vi "SV Multitone SINAD and THD+N (Frequency) (1 Ch).vi"(0 "complex spectrum response":T9={"complex spectrum response"={"f0"=0.0, "df"=1.0, "complex spectrum"=[]}, "spectrum info"={"channel name"="", "description"="", "x-axis units"=0, "spectral info"={"spectrum type"=enum."Power [Magnitude^2]", "linear/dB"=enum."linear", "window"=0, "window size"=0, "FFT size"=0}, "engineering units"=0, "custom label"="", "dB reference [EU]"=0.0, "peak units"=enum."rms", "weighting filter"=0, "spectral density?"=FALSE, "unit label"="", "spectrum skewed?"=FALSE, "complimentary spectrum units"=enum."none"}} {"spectrum info"."x-axis units" items=["Time (s)"=0, "Frequency-CB (Hz)"=1, "Frequency-CPB (Hz)"=1248, "Frequency-Arbitrary (Hz)"=2357, "Quefrency (s)"=2, "Revolutions (rev)"=3, "Order"=4, "Speed (RPM)"=11, "Speed (rad/s)"=21, "Index"=65535]; "spectrum info"."weighting filter" items=["Linear", "A-weighting", "B-weighting", "C-weighting", "ITU-R 468-4", "Dolby", "CCITT", "C-message", "Wb", "Wc", "Wd", "We", "Wf", "Wh", "Wj", "Wk", "Wm", "AES17 20 kHz lowpass", "AES17 40 kHz lowpass", "AES17 20 kHz highpass", "AES17 40 kHz highpass"]; "spectrum info"."dB reference [EU]" format="%.2f"; "spectrum info"."engineering units" items=["custom..."=0, "V"=1, "A"=21, "C"=30, "pC"=31, "s"=32, "-"=29, "Pa"=2, "N"=20, "g"=3, "m/s^2"=4, "m/s"=5, "m"=6, "mm/s"=12, "mm"=13, "micron/s"=14, "micron"=15, "in/s^2"=7, "in/s"=8, "in"=9, "mil/s"=10, "mil"=11, "rad/s^2"=16, "rad/s"=17, "rad"=18, "deg/s^2"=26, "deg/s"=27, "deg"=28, "RPM"=22, "cycle/s^2"=23, "Hz"=24, "cycle"=25, "strain"=19]; "spectrum info"."spectral info"."window" items=["None "=0, "Hanning"=1, "Hamming"=2, "Blackman-Harris"=3, "Exact Blackman"=4, "Blackman"=5, "Flat Top"=6, "4 Term B-Harris "=7, "7 Term B-Harris"=8, "Low Sidelobe"=9, "Force - Exponential"=10, "Gaussian"=62]; "complex spectrum response"."complex spectrum" format="%.2f"; "complex spectrum response"."df" format="%.2f"; "complex spectrum response"."f0" format="%.2f"}, 1 "reference tones":T2(array[cluster]) {"phase (deg)" format="%0.3p"; "amplitude [EU pk]" format="%0.3p"; "frequency [Hz]" format="%0.3p"}, 2 "frequency range":T11={"start frequency"=-1.0, "stop frequency"=-1.0} {"stop frequency" format="%.2f"; "start frequency" format="%.2f"}, 3 "advanced span [Hz]":dbl=-1.0 format="%.2f", 5 "error in (no error)":errorcluster, 6 "desired units":T12={"SINAD"=enum."dB", "THD+N"=enum."dB", "response level"=enum."EU rms", "noise and distortion level"=enum."EU rms"}) -> (12 "unit labels":T10, 14 "complex spectrum response":T9={"complex spectrum response"={"f0"=0.0, "df"=1.0, "complex spectrum"=[]}, "spectrum info"={"channel name"="", "description"="", "x-axis units"=0, "spectral info"={"spectrum type"=enum."Power [Magnitude^2]", "linear/dB"=enum."linear", "window"=0, "window size"=0, "FFT size"=0}, "engineering units"=0, "custom label"="", "dB reference [EU]"=0.0, "peak units"=enum."rms", "weighting filter"=0, "spectral density?"=FALSE, "unit label"="", "spectrum skewed?"=FALSE, "complimentary spectrum units"=enum."none"}} {"spectrum info"."x-axis units" items=["Time (s)"=0, "Frequency-CB (Hz)"=1, "Frequency-CPB (Hz)"=1248, "Frequency-Arbitrary (Hz)"=2357, "Quefrency (s)"=2, "Revolutions (rev)"=3, "Order"=4, "Speed (RPM)"=11, "Speed (rad/s)"=21, "Index"=65535]; "spectrum info"."weighting filter" items=["Linear", "A-weighting", "B-weighting", "C-weighting", "ITU-R 468-4", "Dolby", "CCITT", "C-message", "Wb", "Wc", "Wd", "We", "Wf", "Wh", "Wj", "Wk", "Wm", "AES17 20 kHz lowpass", "AES17 40 kHz lowpass", "AES17 20 kHz highpass", "AES17 40 kHz highpass"]; "spectrum info"."dB reference [EU]" format="%.2f"; "spectrum info"."engineering units" items=["custom..."=0, "V"=1, "A"=21, "C"=30, "pC"=31, "s"=32, "-"=29, "Pa"=2, "N"=20, "g"=3, "m/s^2"=4, "m/s"=5, "m"=6, "mm/s"=12, "mm"=13, "micron/s"=14, "micron"=15, "in/s^2"=7, "in/s"=8, "in"=9, "mil/s"=10, "mil"=11, "rad/s^2"=16, "rad/s"=17, "rad"=18, "deg/s^2"=26, "deg/s"=27, "deg"=28, "RPM"=22, "cycle/s^2"=23, "Hz"=24, "cycle"=25, "strain"=19]; "spectrum info"."spectral info"."window" items=["None "=0, "Hanning"=1, "Hamming"=2, "Blackman-Harris"=3, "Exact Blackman"=4, "Blackman"=5, "Flat Top"=6, "4 Term B-Harris "=7, "7 Term B-Harris"=8, "Low Sidelobe"=9, "Force - Exponential"=10, "Gaussian"=62]; "complex spectrum response"."complex spectrum" format="%.2f"; "complex spectrum response"."df" format="%.2f"; "complex spectrum response"."f0" format="%.2f"}, 15 "SINAD":dbl format="%.2f", 16 "THD+N":dbl format="%.2f", 18 "levels":T1 {"noise and distortion" format="%.2f"; "response" format="%.2f"}, 19 "error out":errorcluster)   [LabVIEW 2017, in "SoundVib_Multitone.lvlib"]
doc: "Performs a total harmonic distortion plus noise (THD+N) analysis, including measuring the fundamental tone, and returns the detected fundamental frequency, detected fundamental amplitude, and THD+N. Signal in noise and distortion (SINAD) is the negative of THD+N in dB. Wire data to the<B> scaled signal [EU]</B> input to determine the polymorphic instance to use or manually select the instance.\n\nThe following formula calculates THD+N:\n\nTHD+N = sqrt(H^2 + N^2) / sqrt(F^2 + N^2 + H^2)\n\nwhere H is the harmonic RMS level, N is the noise RMS level, and F is the fundamental tone RMS level."
uses:
  <vilib>/addons/Sound and Vibration/svt_Multitone Distortion/SoundVib_Multitone.lvlib
  <vilib>/addons/_NISVFA/_Shared subVIs/Controls/svc_Spectrum Info.ctl
  <vilib>/addons/_NISVFA/_Shared subVIs/Controls/svc_X-Axis Units.ctl
  <vilib>/addons/_NISVFA/_Shared subVIs/Controls/svc_Spectrum Type.ctl
  <vilib>/addons/_NISVFA/_Shared subVIs/Controls/svc_Engineering Units Text Ring.ctl
  <vilib>/addons/_NISVFA/_Shared subVIs/Controls/svc_Weighting Filter Text Ring.ctl
  <vilib>/addons/_NISVFA/_Shared subVIs/Controls/svc_Complimentary Spectrum Units.ctl
  <vilib>/addons/_NISVFA/_Spectrum Processing/SVPO Power in Band (Complex) (1 Ch).vi
  <vilib>/Analysis/BLAS.llb/nrm2 - Vector 2-Norm.vi
  <vilib>/Analysis/BLAS.llb/dznrm2 - Vector 2-Norm (CDB).vi
  <vilib>/addons/_NISVFA/_Shared subVIs/Common/svc_Convert Start and Stop to Start Index and Length.vi
  <vilib>/addons/_NISVFA/_Shared subVIs/Common/svc_Window Parameters.vi
  <vilib>/addons/_NISVFA/_Spectrum Processing/subVIs/svfa_Spectrum Info Window to windowTd Type Def.vi
  <vilib>/addons/_NISVFA/_Spectrum Processing/SVFA Get Spectrum Subset (Complex) (1 Ch).vi
  <vilib>/addons/Sound and Vibration/svt_Distortion/SoundVib_Distortion.lvlib
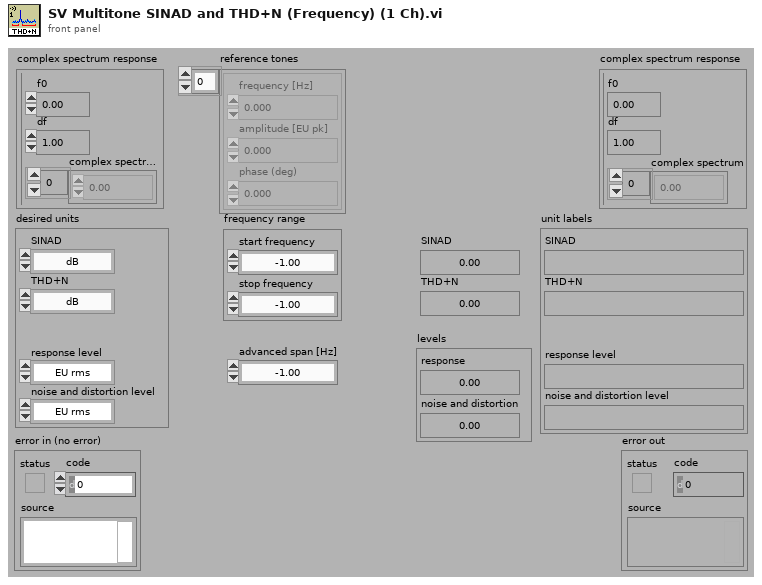
[diagram p1: front panel]
types:
  T1 = cluster{"response":dbl, "noise and distortion":dbl}
  T2 = cluster{"frequency [Hz]":dbl, "amplitude [EU pk]":dbl, "phase (deg)":dbl}[]
  T3 = typedef "svc_Spectrum Info.ctl" = cluster{"channel name":string, "description":string, "x-axis units":T4, "spectral info":cluster{"spectrum type":T5, "linear/dB":enum16{"linear", "dB"}, "window":u16, "window size":i32, "FFT size":i32}, "engineering units":T6, "custom label":string, "dB reference [EU]":dbl, "peak units":enum16{"rms", "peak", "peak-peak"}, "weighting filter":T7, "spectral density?":bool, "unit label":string, "spectrum skewed?":bool, "complimentary spectrum units":T8}
  T4 = typedef "svc_X-Axis Units.ctl" = u16
  T5 = typedef "svc_Spectrum Type.ctl" = enum16{"FFT Spectrum [complex]", "Amplitude [Magnitude]", "Power [Magnitude^2]", "Cross Spectrum [complex]", "Frequency Response [Complex]"}
  T6 = typedef "svc_Engineering Units Text Ring.ctl" = u16
  T7 = typedef "svc_Weighting Filter Text Ring.ctl" = u16
  T8 = typedef "svc_Complimentary Spectrum Units.ctl" = enum16{"none", "radians", "degrees", "cycles", "imaginary"}
  T9 = cluster{"complex spectrum response":cluster{"f0":dbl, "df":dbl, "complex spectrum":cdb[]}, "spectrum info":T3}
  T10 = cluster{"SINAD":string, "THD+N":string, "response level":string, "noise and distortion level":string}
  T11 = cluster{"start frequency":dbl, "stop frequency":dbl}
  T12 = cluster{"SINAD":enum16{"dB", "linear ratio", "%"}, "THD+N":enum16{"dB", "linear ratio", "%"}, "response level":enum16{"EU^2 rms", "EU rms", "dB", "dBc", "dBV", "dBu", "dBm"}, "noise and distortion level":enum16{"EU^2 rms", "EU rms", "dB", "dBc", "dBV", "dBu", "dBm"}}
  T13 = enum32{"none", "input signal", "detected signal", "residual signal"}
  T14 = enum16{"EU^2 rms", "EU rms", "dB", "dBc", "dBV", "dBu", "dBm"}
  T15 = cluster{"complex spectrum subset":cluster{"x0":dbl, "dx":dbl, "complex array":cdb[]}, "spectrum info":T3}
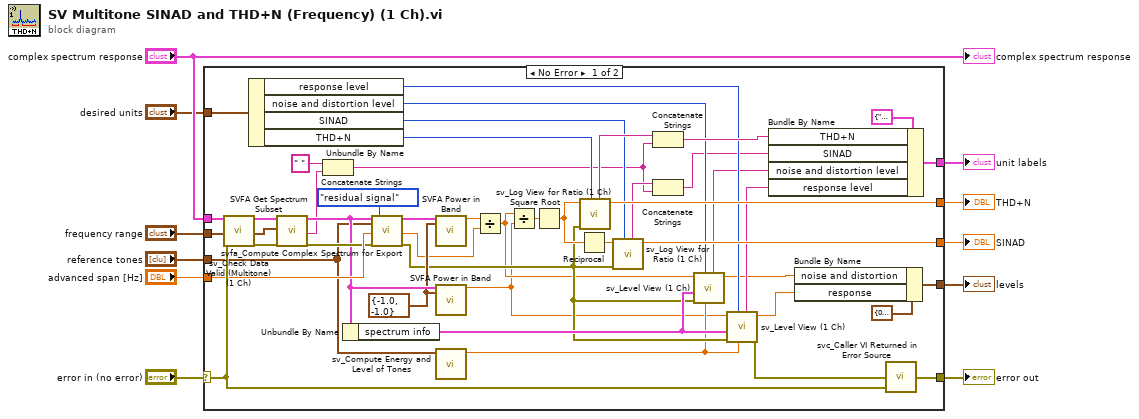
[diagram p0: block diagram]
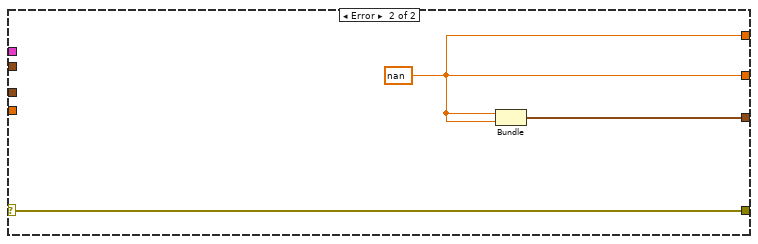
[diagram p2: hidden frame]
diagram:
  n1 = case shown="No Error" "error in (no error)" {
    selector: "error in (no error)" -> [w49 w61]
    tunnel: "complex spectrum response" -> [w51 _]
    tunnel: [w58 w61] -> w10
    tunnel: [w56 w60] -> w9
    tunnel: "frequency range" -> [w50 _]
    tunnel: "desired units" -> [w57 _]
    tunnel: [w54 _] -> w1
    tunnel: "reference tones" -> [w24 _]
    tunnel: "advanced span [Hz]" -> [w48 _]
    tunnel: [w36 w60] -> w3
    tunnel: [w25 w59] -> w2
    frame No Error {
      w41 = cluster{"start":dbl, "stop":dbl} {"start"=-1.0, "stop"=-1.0} ("range")
      n2 = call <vilib>:"sv_Check Data Valid (Multitone) (1 Ch).vi"("complex spectrum"=w51, "frequency range in [Hz]"=w50, "error in (no error)"=w49) -> ("complex spectrum"=w46:T9, "frequency range out [Hz]"=w47:cluster{"start":dbl, "stop":dbl}, "error out"=w45:errorcluster)  [unwired: 14 in]
      n3 = Unbundle By Name(w57) -> ("response level"=w33:T14, "noise and distortion level"=w34:T14, "SINAD"=w40:enum16{"dB", "linear ratio", "%"}, "THD+N"=w55:enum16{"dB", "linear ratio", "%"})
      n4 = call-poly <vilib>:"SVFA Get Spectrum Subset.vi"("complex spectrum"=w46, "range"=w47, "error in (no error)"=w45) -> ("complex spectrum subset"=w42:T15, "range label"=w18:string, "error out"=w44:errorcluster)  [unwired: 13 in, 1 out]
      n5 = Concatenate Strings(" " ("string"), w18) -> (w20:string)
      n6 = Unbundle By Name(w42) -> ("spectrum info"=w35:T3)
      n7 = call <vilib>:"svfa_Compute Complex Spectrum for Export.vi"("complex spectrum in"=w42, "tones"=w24, "advanced span [Hz]"=w48, "error in"=w44, "export signals"=T13."residual signal") -> ("complex spectrum out"=w43:T9, "residual bandwidth ratio"=w15:dbl, "error out"=w32:errorcluster)  [unwired: 12 in]
      n8 = call-poly <vilib>:"SVFA Power in Band.vi"("complex spectrum"=w43, "range"=w41) -> ("power in band [EU^2 rms]"=w16:dbl)  [unwired: 17 in]
      n9 = call-poly <vilib>:"SVFA Power in Band.vi"("complex spectrum"=w42, "range"=w41) -> ("power in band [EU^2 rms]"=w13:dbl)  [unwired: 17 in]
      n10 = call <vilib>:"sv_Compute Energy and Level of Tones.vi"("reference tones"=w24) -> ("energy level [EU^2 rms]"=w23:dbl)  [unwired: 9 in, 1 out]
      n11 = Divide(x=w16, y=w15) -> (x/y=w14:dbl)
      n12 = Divide(x=w14, y=w13) -> (x/y=w12:dbl)
      n13 = Square Root(x=w12) -> (sqrt(x)=w39:dbl)
      n14 = Reciprocal(x=w39) -> (1/x=w38:dbl)
      n15 = call <vilib>:"sv_Log View for Ratio (1 Ch).vi"("ratio units"=w55, "error in (no error)"=w32, "linear ratio"=w39) -> ("converted ratio"=w56:dbl, "unit label"=w53:string)  [unwired: 6 in, 1 out]
      n16 = call <vilib>:"sv_Log View for Ratio (1 Ch).vi"("ratio units"=w40, "error in (no error)"=w32, "linear ratio"=w38) -> ("converted ratio"=w36:dbl, "unit label"=w37:string)  [unwired: 6 in, 1 out]
      n17 = Concatenate Strings(w53, w20) -> (w52:string)
      n18 = Concatenate Strings(w37, w20) -> (w31:string)
      n19 = call <vilib>:"sv_Level View (1 Ch).vi"("carrier level [EU^2 rms]"=w23, "desired units"=w34, "error in (no error)"=w32, "spectrum info"=w35, "level [EU^2 rms]"=w14) -> ("converted level"=w27:dbl, "unit label"=w30:string)  [unwired: 4 in, 1 out]
      n20 = call <vilib>:"sv_Level View (1 Ch).vi"("carrier level [EU^2 rms]"=w23, "desired units"=w33, "error in (no error)"=w32, "spectrum info"=w35, "level [EU^2 rms]"=w13) -> ("error out"=w19:errorcluster, "converted level"=w26:dbl, "unit label"=w29:string)  [unwired: 4 in]
      n21 = Bundle By Name(cluster=T10 {"SINAD"="", "THD+N"="", "response level"="", "noise and distortion level"=""} ("unit labels"), "THD+N"=w52, "SINAD"=w31, "noise and distortion level"=w30, "response level"=w29) -> (w54:T10)
      n22 = Bundle By Name(cluster=T1 {"response"=0.0, "noise and distortion"=0.0} ("levels"), "noise and distortion"=w27, "response"=w26) -> (w25:T1)
      n23 = call <vilib>:"svc_Caller VI Returned in Error Source.vi"("warning input to caller"=w49, "error in (no error)"=w19) -> ("error out"=w58:errorcluster)  [unwired: 3 in]
    }
    frame Error {
      w60 = nan ("SINAD")
      n24 = Bundle("SINAD"=w60, "SINAD"=w60) -> (w59:cluster{"SINAD":dbl, "SINAD":dbl})  [unwired: 1 in]
    }
  }
  "error out" <- w10
  "THD+N" <- w9
  "unit labels" <- w1
  "SINAD" <- w3
  "levels" <- w2
  "complex spectrum response" <- "complex spectrum response"
